vi "edittest extract record keys.vi"(6 "User Record":T1, 7 "Template Keys In (empty)":T2, 8 "error in (no error)":errorcluster, 10 "Sequence Record":T3, 11 "Connection Refnum":T4) -> (0 "error out":errorcluster, 3 "Connection Refnum":T4, 5 "Template Keys Out":T2)   [LabVIEW 2011]
uses:
  Summitek EXT/ODBC/SQL Controls/Connection Refnum.ctl
  server/database/Sequences/Sequence Record.ctl
  ITK EXT/utils/keyedarr.llb/Keyed Array.ctl
  server/database/Users/User Record.ctl
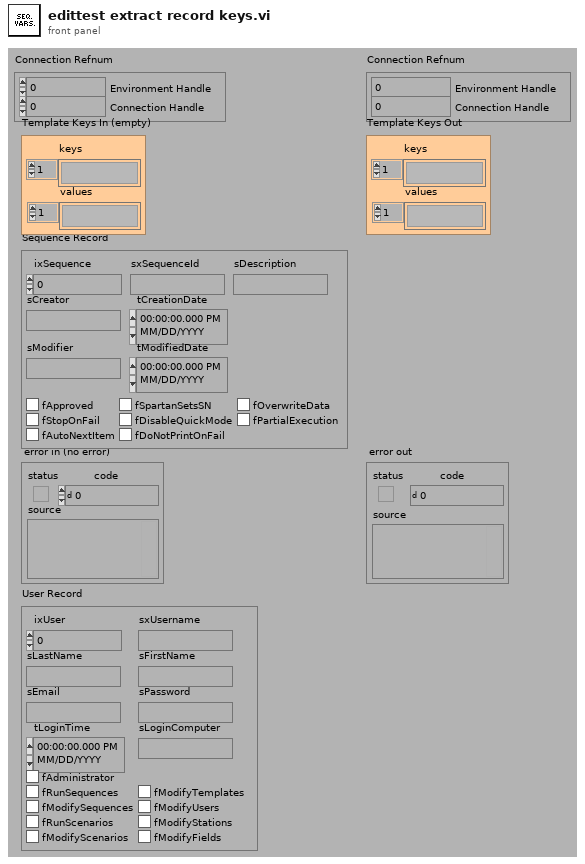
[diagram p1: front panel]
types:
  T1 = typedef "User Record.ctl" = cluster{"ixUser":i32, "sxUsername":string, "sLastName":string, "sFirstName":string, "sEmail":string, "sPassword":string, "tLoginTime":timestamp, "sLoginComputer":string, "fAdministrator":bool, "fRunSequences":bool, "fModifySequences":bool, "fRunScenarios":bool, "fModifyScenarios":bool, "fModifyTemplates":bool, "fModifyUsers":bool, "fModifyStations":bool, "fModifyFields":bool}
  T2 = typedef "Keyed Array.ctl" = cluster{"keys":string[], "values":string[]}
  T3 = typedef "Sequence Record.ctl" = cluster{"ixSequence":i32, "sxSequenceId":string, "sDescription":string, "sCreator":string, "tCreationDate":timestamp, "sModifier":string, "tModifiedDate":timestamp, "fApproved":bool, "fSpartanSetsSN":bool, "fOverwriteData":bool, "fStopOnFail":bool, "fDisableQuickMode":bool, "fPartialExecution":bool, "fAutoNextItem":bool, "fDoNotPrintOnFail":bool}
  T4 = typedef "Connection Refnum.ctl" = cluster{"Environment Handle":i32, "Connection Handle":i32}
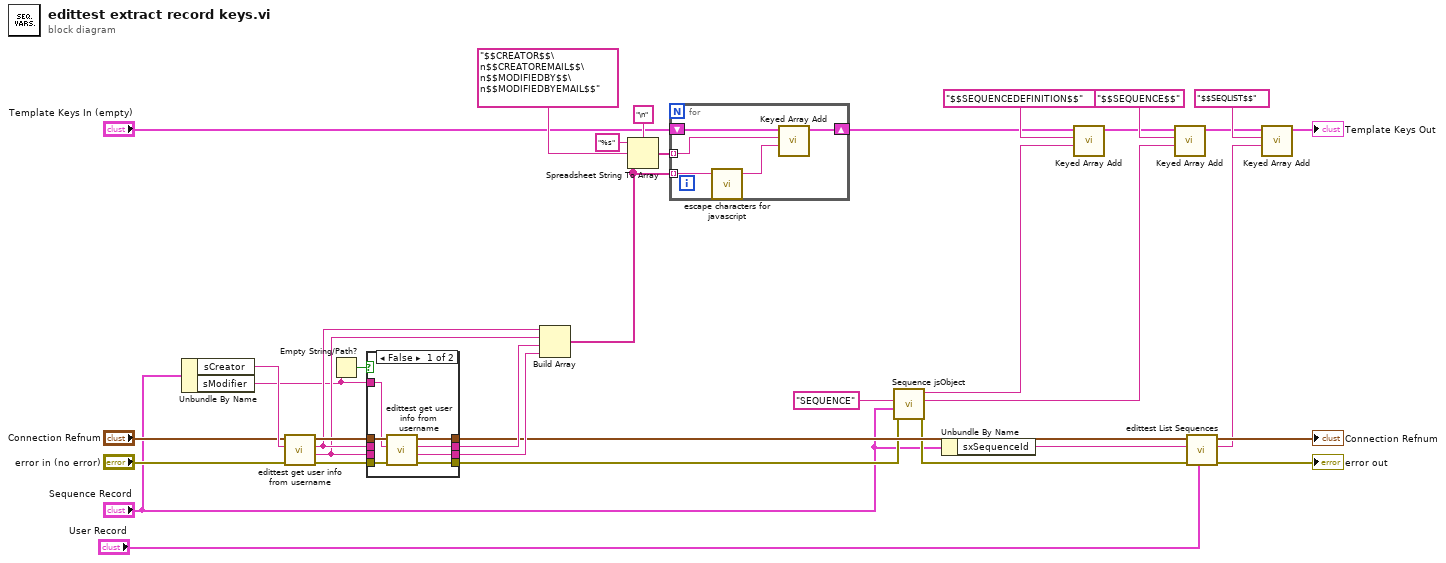
[diagram p0: block diagram]
diagram:
  n1 = Unbundle By Name("Sequence Record") -> ("sCreator"=w36:string, "sModifier"=w20:string)
  n2 = call "edittest get user info from username.vi"("error in (no error)"="error in (no error)", "Username (\"\")"=w36, "Connection Refnum"="Connection Refnum") -> ("error out"=w34:errorcluster, "Email"=w31:string, "First Last"=w32:string, "Connection Refnum"=w35:T4)  [unwired: 5 out]
  n3 = Empty String/Path?(string/path=w20) -> (empty?=w33:bool)
  n4 = case shown="False" w33 {
    tunnel: w35 -> [w43 w47]
    tunnel: w34 -> [w42 w46]
    tunnel: w20 -> [w41 _]
    tunnel: w32 -> [_ w45]
    tunnel: w31 -> [_ w44]
    tunnel: [w40 w47] -> w18
    tunnel: [w39 w46] -> w7
    tunnel: [w38 w45] -> w30
    tunnel: [w37 w44] -> w29
    frame False {
      n5 = call "edittest get user info from username.vi"("error in (no error)"=w42, "Username (\"\")"=w41, "Connection Refnum"=w43) -> ("error out"=w39:errorcluster, "Email"=w37:string, "First Last"=w38:string, "Connection Refnum"=w40:T4)  [unwired: 5 out]
    }
    frame True {
    }
  }
  n6 = Build Array(w32, w31, w30, w29) -> (w24:string[])
  n7 = Spreadsheet String To Array(delimiter (Tab)="\n", format string="%s", spreadsheet string="$$CREATOR$$\n$$CREATOREMAIL$$\n$$MODIFIEDBY$$\n$$MODIFIEDBYEMAIL$$", array type (2D Dbl)=w24) -> (array=w25:string[])
  n8 = for {
    shift-right: [w51] -> w1
    shift-left: "Template Keys In (empty)" -> [w52]
    tunnel: w25 -> [w50] mode=indexing
    tunnel: w24 -> [w49] mode=indexing
    n9 = call "escape characters for javascript.vi"("String (\"\")"=w49) -> ("escaped String"=w48:string)  [unwired: 4 out]
    n10 = call "Keyed Array Add.vi"("value"=w48, "key"=w50, "array in"=w52) -> ("array out"=w51:T2)  [unwired: 1 in, 3 out]
  }
  n11 = call "Sequence jsObject.vi"("error in (no error)"=w7, "Sequence Record (empty)"="Sequence Record", "Sequence jsObject Name (\"\")"="SEQUENCE" ("Scenario jsObject Name (\"\")")) -> ("error out"=w8:errorcluster, "Sequence jsObject"=w4:string, "SEQUENCE jsObject Definition"=w5:string)  [unwired: 1 in, 5 out]
  n12 = Unbundle By Name("Sequence Record") -> ("sxSequenceId"=w2:string)
  n13 = call "Keyed Array Add.vi"("value"=w5, "key"="$$SEQUENCEDEFINITION$$" ("format string"), "array in"=w1) -> ("array out"=w10:T2)  [unwired: 1 in, 3 out]
  n14 = call "Keyed Array Add.vi"("value"=w4, "key"="$$SEQUENCE$$" ("format string"), "array in"=w10) -> ("array out"=w6:T2)  [unwired: 1 in, 3 out]
  n15 = call "edittest List Sequences.vi"("User Information"="User Record", "error in (no error)"=w8, "sxSequenceId (\"\")"=w2, "Connection Refnum"=w18) -> ("error out"=→"error out":errorcluster, "Sequences List"=w15:string, "Connection Refnum"=→"Connection Refnum":T4)  [unwired: 5 out]
  n16 = call "Keyed Array Add.vi"("value"=w15, "key"="$$SEQLIST$$" ("format string"), "array in"=w6) -> ("array out"=→"Template Keys Out":T2)  [unwired: 1 in, 3 out]
